vi "Step6_0_LowPass.vi"(9 "s_axis_data_tdata":fxp<+/-,24,1>, 10 "s_axis_data_tvalid":bool) -> (1 "m_axis_data_tdata":fxp<+/-,24,2>, 2 "m_axis_data_tvalid":bool, 3 "s_axis_data_tready":bool)   [LabVIEW 2018]
uses:
  <vilib>/rvi/IPIntegrationNode/IPINode_Typedef/niFpgaIPINodeSupportedFamilies.ctl
  <vilib>/rvi/IPIntegrationNode/IPINode_Utilities/niFpgaIPINodeSimCore.vi
  <vilib>/rvi/XilinxIP/XIPIN_XNode/niFpgaXIPIN.xnode
  FIR_Filter_Configuration/FIR Compiler/xsim.dir/FIR_Compiler_3CE652926F5B43F18022D1349C670FA0/xsimk_3CE652926F5B43F18022D1349C670FA0.dll
  <vilib>/rvi/IPIntegrationNode/IPINode_Xnode/niFpgaIPINode.xnode
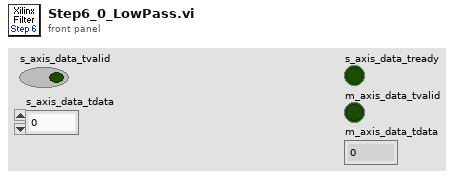
[diagram p1: front panel]
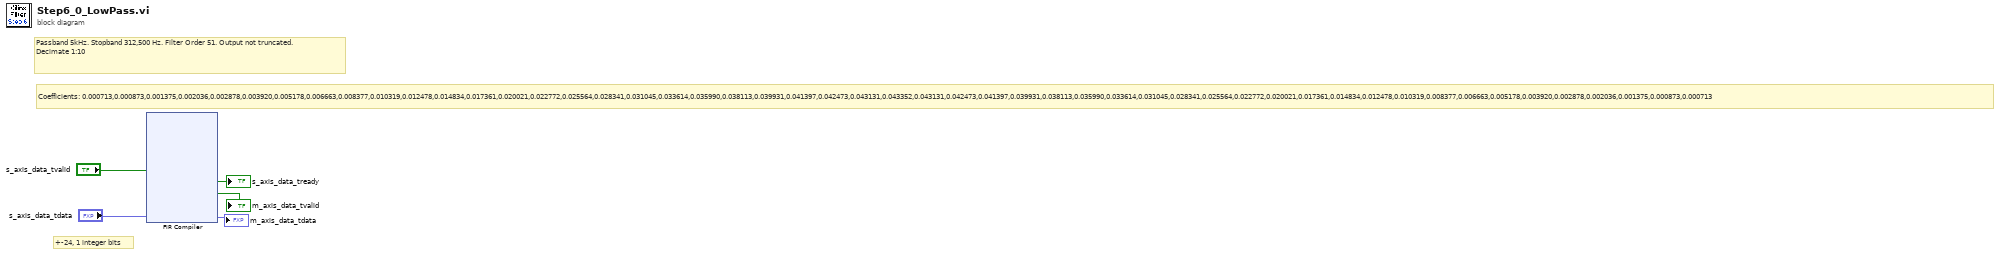
[diagram p0: block diagram]
diagram:
  # "+-24, 1 integer bits"
  # "Coefficients: 0.000713,0.000873,0.001375,0.002036,0.002878,0.003920,0.005178,0.006663,0.008377,0.010319,0.012478,0.014834,0.017361,0.020021,0.022772,0.025564,0.028341,0.031045,0.033614,0.035990,0.038113,0.039931,0.041397,0.042473,0.043131,0.043352,0.043131,0.042473,0.041397,0.039931,0.038113,0.035990,0.033614,0.031045,0.028341,0.025564,0.022772,0.020021,0.017361,0.014834,0.012478,0.010319,0.008377,0.006663,0.005178,0.003920,0.002878,0.002036,0.001375,0.000873,0.000713"
  # "Passband 5kHz. Stopband 312,500 Hz. Filter Order 51. Output not truncated.\nDecimate 1:10"
  n1 = xnode ("FIR Compiler")("s_axis_data_tvalid"="s_axis_data_tvalid", "s_axis_data_tdata"="s_axis_data_tdata") -> ("s_axis_data_tready"=→"s_axis_data_tready":bool, "m_axis_data_tvalid"=→"m_axis_data_tvalid":bool, "m_axis_data_tdata"=→"m_axis_data_tdata":fxp<+/-,24,2>)
